vi "CC Script Execute Step.vi"(8 "error in (no error)":errorcluster, 11 "Script Step":T1={"Action"=enum."Acquire Images", "Data"=variant}) -> (0 "error out":errorcluster)   [LabVIEW 2024]
uses:
  typedefs/CC Script Step.ctl
  typedefs/CC enum Script Action.ctl
  Subsystems/SS typedef cluster Instrument Command Queue Data.ctl
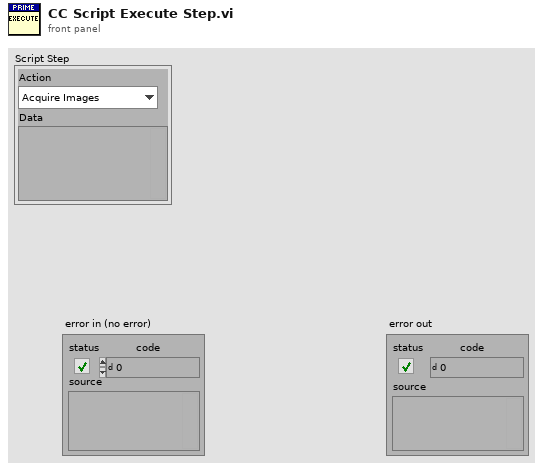
[diagram p1: front panel]
types:
  T1 = typedef "CC Script Step.ctl" = cluster{"Action":T2, "Data":variant}
  T2 = typedef "CC enum Script Action.ctl" = enum16{"Noop", "Define Object", "Define Exposure", "Define Dithering", "Acquire Images", "Set Filter Wheel", "Telescope Home", "Telescope Move", "Telescope RA DEC", "Focus Move Relative", "Focus Move Absolute", "Focus Set Home", "Macro", "Pause", "Ask User", "Define Random Dither"}
  T3 = typedef "SS typedef cluster Instrument Command Queue Data.ctl" = cluster{"Cmd":string, "Parameters":variant}
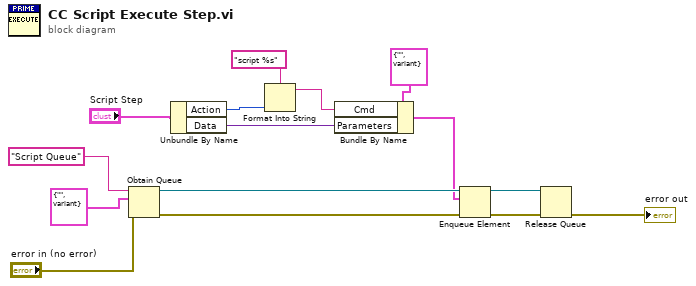
[diagram p0: block diagram]
diagram:
  n1 = Obtain Queue(name (unnamed)="Script Queue", element data type=T3 {"Cmd"="", "Parameters"=variant}, error in (no error)="error in (no error)") -> (queue out=w9:refnum<queue>, error out=w3:errorcluster)  [unwired: 2 in, 1 out]
  n2 = Unbundle By Name("Script Step") -> ("Action"=w11:T2, "Data"=w6:variant)
  n3 = Format Into String(format string="script %s" ("Cmd"), w11) -> (resulting string=w7:string)  [unwired: 2 in, 1 out]
  n4 = Bundle By Name(cluster=T3 {"Cmd"="", "Parameters"=variant} ("element"), "Cmd"=w7, "Parameters"=w6) -> (w5:T3)
  n5 = Enqueue Element(queue=w9, element=w5, error in (no error)=w3) -> (queue out=w1:refnum<queue>, error out=w2:errorcluster)  [unwired: 1 in, 1 out]
  n6 = Release Queue(queue=w1, error in (no error)=w2) -> (error out=→"error out":errorcluster)  [unwired: 1 in, 2 out]
